vi "SetupInterface.vi"(8 "error in (no error)":errorcluster, 11 "AbstractStep in":refnum<class "Measure.lvclass">) -> (0 "error out":errorcluster, 3 "AbstractStep out":refnum<class "Measure.lvclass">)   [LabVIEW 2014, in "Measure.lvclass"]
uses:
  Measure.lvclass
  StepData/Control/MeasureData.ctl
  StepData/StepData.lvclass
panel:
  in  "Log?":bool
  out "Step Name":string
  in  "Sensor No.":i32
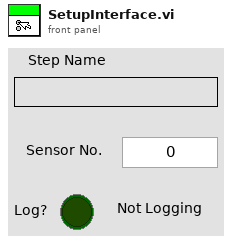
[diagram p1: front panel]
types:
  T1 = typedef "StepData.lvclass/MeasureData.ctl" = cluster{"Sensor No.":i32, "Log?":bool}
  T2 = typedef "StepData.lvclass/AllStepTypeData.ctl" = cluster{"StepName":string, "StepTypeEnum":T3, "MoveData":T4, "MeasureData":T1}
  T3 = typedef "StepData.lvclass/StepTypeEnum.ctl" = enum16{"Move", "Measure"}
  T4 = typedef "StepData.lvclass/MoveData.ctl" = cluster{"Axis":u16, "Position":dbl, "Speed":dbl, "Acc/Dec":dbl, "Mode":u16}
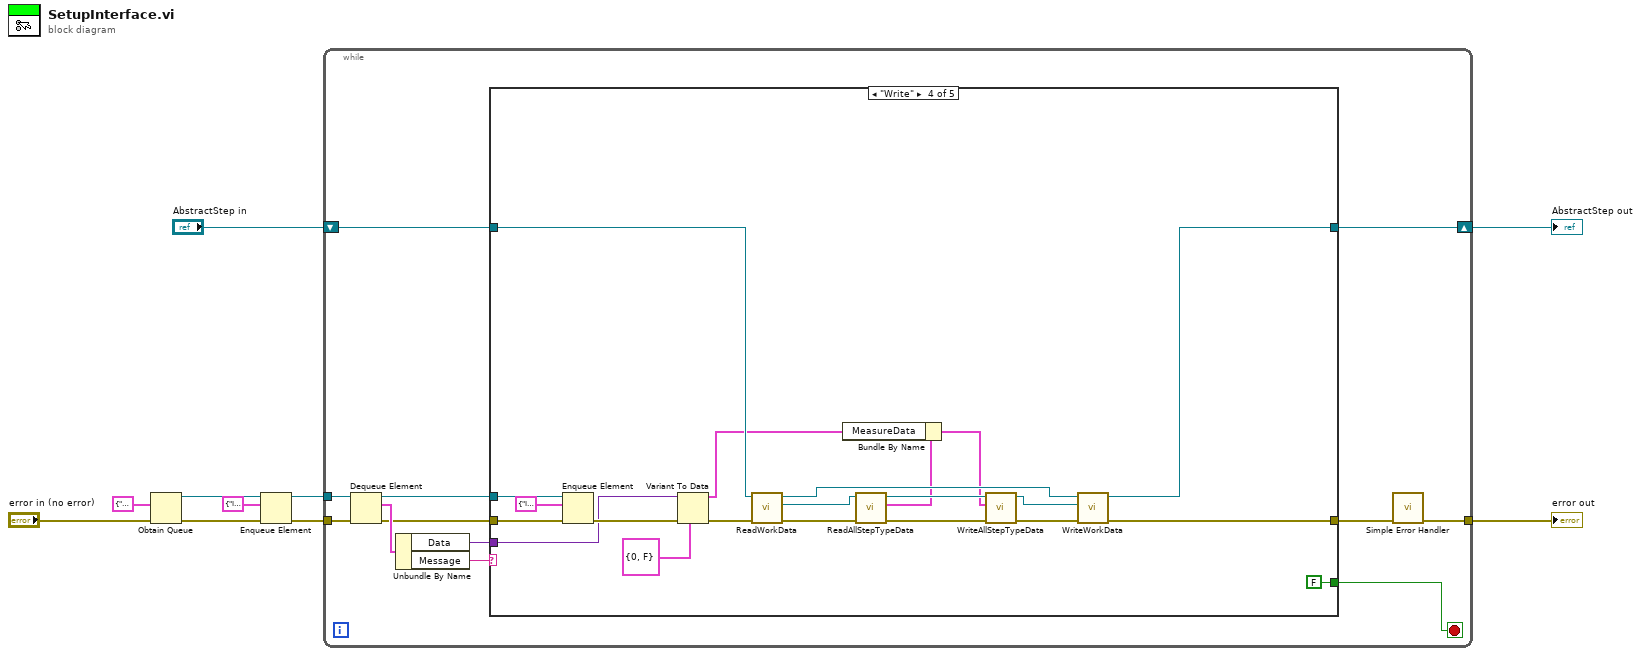
[diagram p0: block diagram]
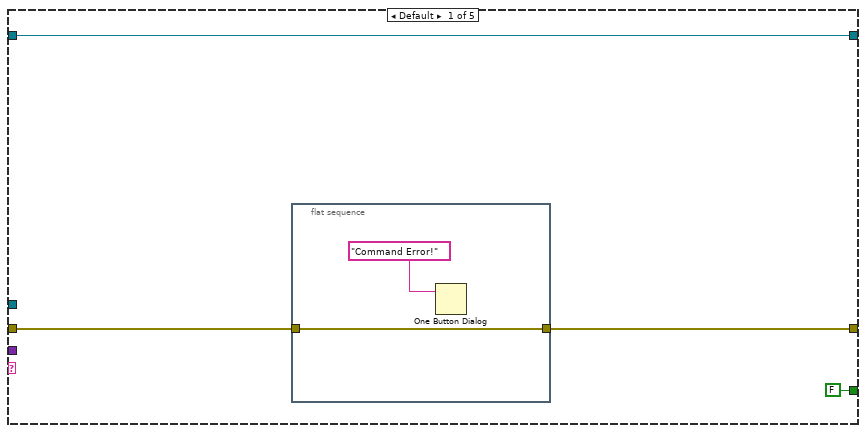
[diagram p2: hidden frame]
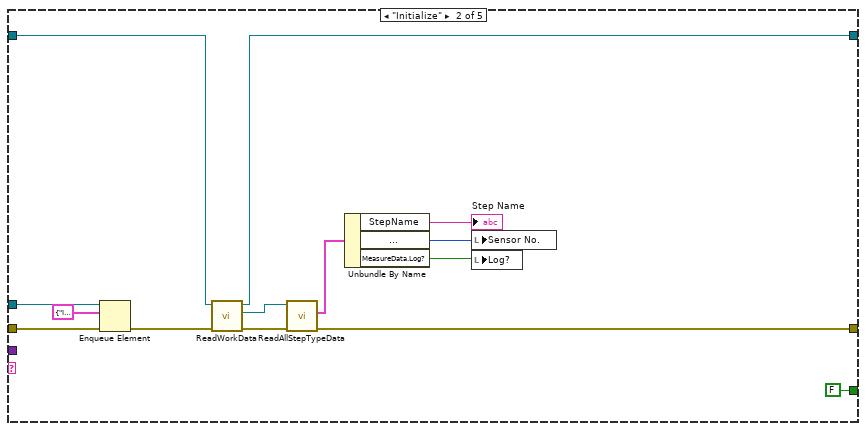
[diagram p3: hidden frame]
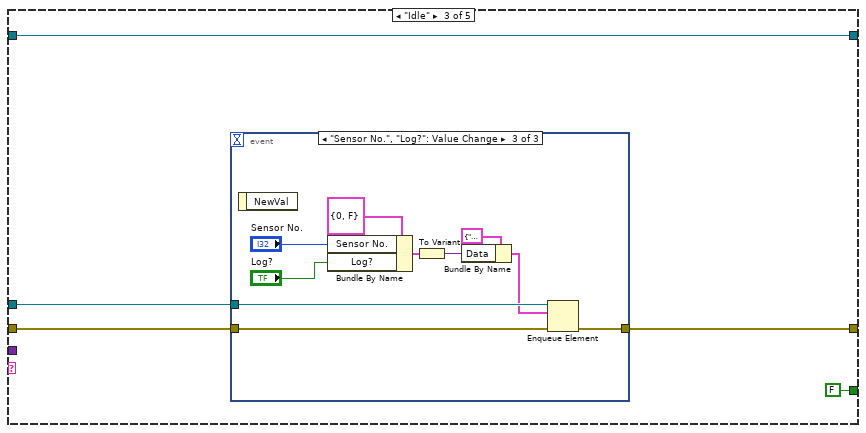
[diagram p4: hidden frame]
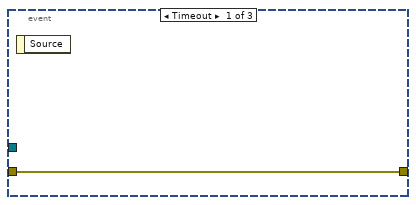
[diagram p5: hidden frame]
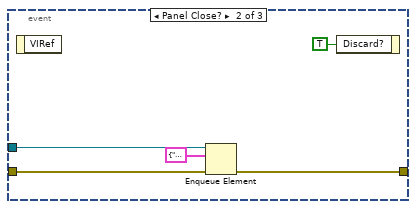
[diagram p6: hidden frame]
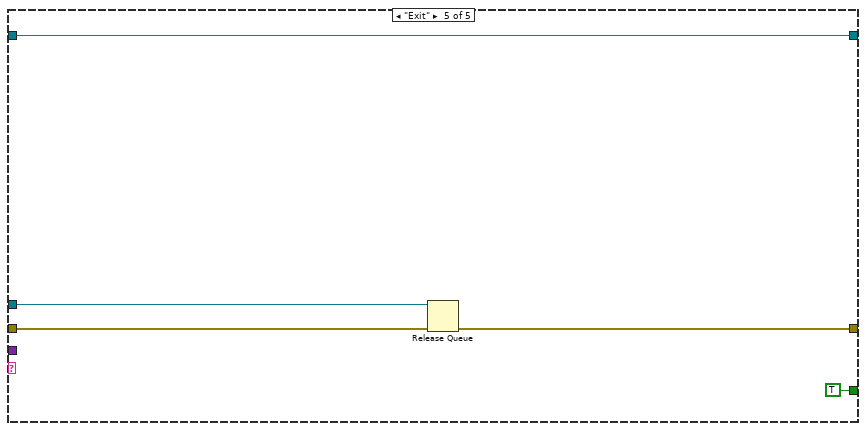
[diagram p7: hidden frame]
diagram:
  n1 = Obtain Queue(element data type=cluster{"Message":string, "Data":variant} {"Message"="", "Data"=variant}, error in (no error)="error in (no error)") -> (queue out=w9:refnum<queue>, error out=w10:errorcluster)  [unwired: 3 in, 1 out]
  n2 = Enqueue Element(queue=w9, element=cluster{"Message":string, "Data":variant} {"Message"="Initialize", "Data"=variant}, error in (no error)=w10) -> (queue out=w6:refnum<queue>, error out=w5:errorcluster)  [unwired: 1 in, 1 out]
  n3 = while {
    tunnel: w6 -> [w22]
    tunnel: w5 -> [w21]
    tunnel: [w14] -> w3
    shift-right: [w12] -> w1
    shift-left: "AbstractStep in" -> [w13]
    stop <- w15 stop-if-true
    n4 = Dequeue Element(queue=w22, error in (no error)=w21) -> (queue out=w16:refnum<queue>, element=w20:cluster{"Message":string, "Data":variant}, error out=w18:errorcluster)  [unwired: 1 in, 1 out]
    n5 = Unbundle By Name(w20) -> ("Data"=w11:variant, "Message"=w19:string)
    n6 = case shown="\"Write\"" w19 {
      tunnel: w18 -> [w26 w42 w46 w84 w88]
      tunnel: [w25 w34 w45 w73 w86] -> w17
      tunnel: w16 -> [_ w41 w47 w83 w87]
      tunnel: [FALSE FALSE FALSE FALSE TRUE] -> w15
      tunnel: w13 -> [w23 w37 w43 w80 w85]
      tunnel: [w23 w36 w43 w79 w85] -> w12
      tunnel: w11 -> [_ _ _ w68 _]
      frame Default {
        n7 = flat-sequence {
          tunnel: w26 -> [w28]
          tunnel: [w28] -> w25
          frame #0 {
            n8 = One Button Dialog(message="Command Error!") -> ()  [unwired: 1 in, 1 out]
          }
        }
      }
      frame "Initialize" {
        n9 = Enqueue Element(queue=w41, element=cluster{"Message":string, "Data":variant} {"Message"="Idle", "Data"=variant}, error in (no error)=w42) -> (error out=w38:errorcluster)  [unwired: 1 in, 2 out]
        n10 = call-dynamic "ReadWorkData.vi"("error in (no error)"=w38, "AbstractStep in"=w37) -> ("error out"=w35:errorcluster, "StepData.lvclass"=w33:refnum<class "StepData.lvclass">, "AbstractStep out"=w36:refnum<class "Measure.lvclass">)  [unwired: 7 in]
        n11 = call "ReadAllStepTypeData.vi"("error in (no error)"=w35, "StepData.lvclass In"=w33) -> ("error out"=w34:errorcluster, "AllStepTypeData"=w32:T2)  [unwired: 7 in, 1 out]
        n12 = Unbundle By Name(w32) -> ("StepName"=→"Step Name":string, "MeasureData.Sensor No."=w30:i32, "MeasureData.Log?"=w29:bool)
        n13 = local write "Sensor No."(w30) -> ()
        n14 = local write "Log?"(w29) -> ()
      }
      frame "Idle" {
        n15 = event shown="[2] \"Sensor No.\", \"Log?\": Value Change" {
          selector: _ -> [_ _ _]
          dyn-events: _ -> [_ _ _]
          timeout: _ -> [_ _ _]
          tunnel: w47 -> [_ w50 w62]
          tunnel: w46 -> [w48 w52 w63]
          tunnel: [w48 w51 w61] -> w45
          event Timeout {
            n16 = event-data() -> ()  [unwired: 1 in, 1 out]
          }
          event Panel Close? {
            n17 = event-data() -> ()  [unwired: 1 in, 1 out]
            n18 = Enqueue Element(queue=w50, element=cluster{"Message":string, "Data":variant} {"Message"="Exit", "Data"=variant}, error in (no error)=w52) -> (error out=w51:errorcluster)  [unwired: 1 in, 2 out]
            n19 = event-data("Discard?"=TRUE) -> ()  [unwired: 1 in, 1 out]
          }
          event "Sensor No.", "Log?": Value Change {
            n20 = event-data() -> ()  [unwired: 1 in, 1 out]
            n21 = Bundle By Name(cluster=T1 {"Sensor No."=0, "Log?"=FALSE} ("MeasureData"), "Sensor No."="Sensor No.", "Log?"="Log?") -> (w56:T1)
            n22 = To Variant(anything=w56) -> (Variant=w55:variant)
            n23 = Bundle By Name(cluster=cluster{"Message":string, "Data":variant} {"Message"="Write", "Data"=variant} ("element"), "Data"=w55) -> (w54:cluster{"Message":string, "Data":variant})
            n24 = Enqueue Element(queue=w62, element=w54, error in (no error)=w63) -> (error out=w61:errorcluster)  [unwired: 1 in, 2 out]
          }
        }
      }
      frame "Write" {
        n25 = Enqueue Element(queue=w83, element=cluster{"Message":string, "Data":variant} {"Message"="Idle", "Data"=variant}, error in (no error)=w84) -> (error out=w70:errorcluster)  [unwired: 1 in, 2 out]
        n26 = Variant To Data(error in=w70, type=T1 {"Sensor No."=0, "Log?"=FALSE} ("MeasureData"), Variant=w68) -> (data=w66:T1, error out=w69:errorcluster)
        n27 = call-dynamic "ReadWorkData.vi"("error in (no error)"=w69, "AbstractStep in"=w80) -> ("error out"=w75:errorcluster, "StepData.lvclass"=w78:refnum<class "StepData.lvclass">, "AbstractStep out"=w72:refnum<class "Measure.lvclass">)  [unwired: 7 in]
        n28 = call "ReadAllStepTypeData.vi"("error in (no error)"=w75, "StepData.lvclass In"=w78) -> ("error out"=w74:errorcluster, "AllStepTypeData"=w71:T2, "StepData.lvclass Out"=w77:refnum<class "StepData.lvclass">)  [unwired: 7 in]
        n29 = Bundle By Name(cluster=w71, "MeasureData"=w66) -> (w64:T2)
        n30 = call "WriteAllStepTypeData.vi"("error in (no error)"=w74, "AllStepTypeData"=w64, "StepData.lvclass In"=w77) -> ("error out"=w65:errorcluster, "StepData.lvclass Out"=w76:refnum<class "StepData.lvclass">)  [unwired: 7 in]
        n31 = call-dynamic "WriteWorkData.vi"("error in (no error)"=w65, "StepData.lvclass"=w76, "AbstractStep in"=w72) -> ("error out"=w73:errorcluster, "AbstractStep out"=w79:refnum<class "Measure.lvclass">)  [unwired: 7 in]
      }
      frame "Exit" {
        n32 = Release Queue(queue=w87, error in (no error)=w88) -> (error out=w86:errorcluster)  [unwired: 1 in, 2 out]
      }
    }
    n33 = call <vilib>:"Simple Error Handler.vi"("error in (no error)"=w17) -> ("error out"=w14:errorcluster)  [unwired: 4 in, 4 out]
  }
  "error out" <- w3
  "AbstractStep out" <- w1
